vi "write floor encoder count.vi"(8 "Next Floor":string="Ground Floor: ", 9 "Current Floor":T1, 10 "Counter Value in":i32) -> (1 "error out":errorcluster)   [LabVIEW 2017]
uses:
  Working Demo Phase/Current Floor.ctl
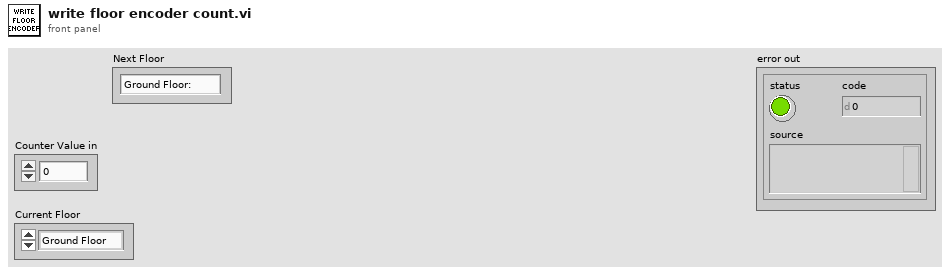
[diagram p1: front panel]
types:
  T1 = typedef "Current Floor.ctl" = enum16{"Ground Floor", "Floor 1", "Floor 2"}
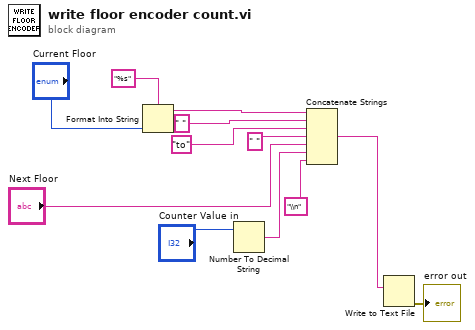
[diagram p0: block diagram]
diagram:
  n1 = Format Into String(format string="%s", "Current Floor") -> (resulting string=w9:string)  [unwired: 2 in, 1 out]
  n2 = Number To Decimal String(number="Counter Value in") -> (decimal integer string=w2:string)  [unwired: 1 in]
  n3 = Concatenate Strings(w9, " " ("string"), "to" ("string"), " " ("string"), "Next Floor", w2, "\\n" ("string")) -> (w6:string)
  n4 = Write to Text File(text=w6) -> (error out=→"error out":errorcluster)  [unwired: 3 in, 2 out]
